vi "Create XML File.vi"() -> ()   [LabVIEW 2016]
uses:
  Array Device Info.ctl
  Device Info.ctl
  Globals.vi
panel:
  in  "array of devices":T1
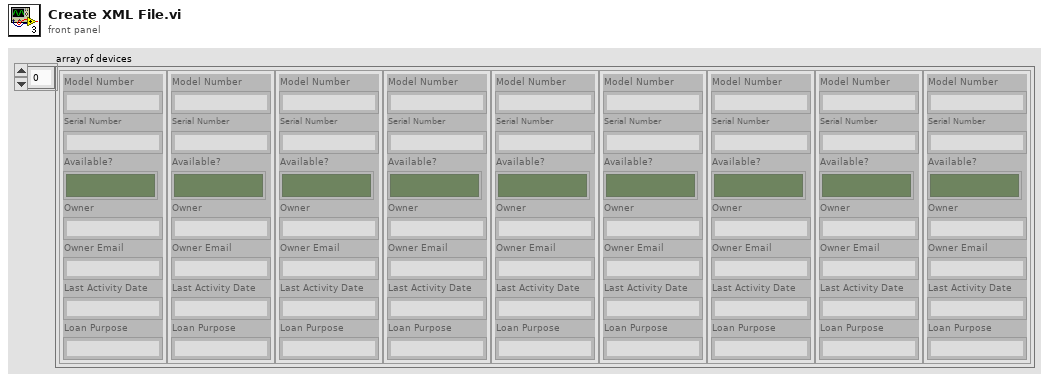
[diagram p1: front panel]
types:
  T1 = typedef "Array Device Info.ctl" = T2[]
  T2 = typedef "Device Info.ctl" = cluster{"Model Number":string, "Serial Number":string, "Available?":bool, "Owner":string, "Owner Email":string, "Last Activity Date":string, "Loan Purpose":string}
  T3 = enum16{"open", "replace", "create", "open or create", "replace or create", "replace or create with confirmation"}
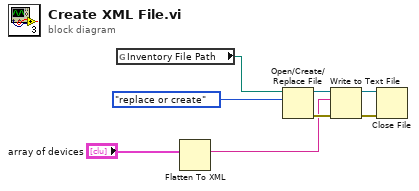
[diagram p0: block diagram]
diagram:
  n1 = global read "Globals.vi" "Inventory File Path"() -> (w2:path)
  n2 = Flatten To XML(anything="array of devices") -> (xml string=w3:string)
  n3 = Open/Create/Replace File(file path (use dialog)=w2, operation (0:open)=T3."replace or create") -> (refnum out=w4:refnum<file>, error out=w7:errorcluster)  [unwired: 4 in, 1 out]
  n4 = Write to Text File(file (use dialog)=w4, text=w3, error in=w7) -> (refnum out=w5:refnum<file>, error out=w6:errorcluster)  [unwired: 1 in, 1 out]
  n5 = Close File(refnum=w5, error in=w6) -> ()  [unwired: 2 out]
